vi "user32_BringWindowToTop.vi"(0 "hWnd":u32, 11 "错误输入（无错误）":errorcluster) -> (4 "dup hWnd":u32, 6 "success?":bool, 15 "错误输出":errorcluster)   [LabVIEW 2011]
doc: "该函数将指定的窗口设置到Z序的顶部。如果窗口为顶层窗口，则该窗口被激活；如果窗口为子窗口，则相应的顶级父窗口被激活。"
uses:
  user32.dll
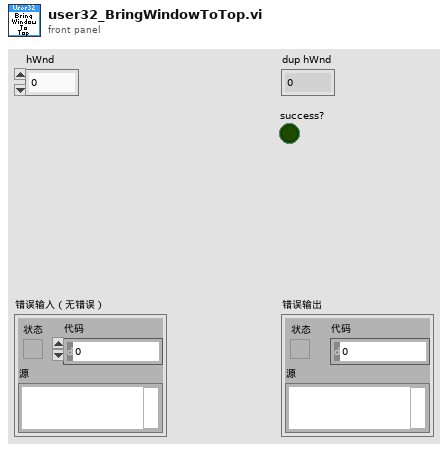
[diagram p1: front panel]
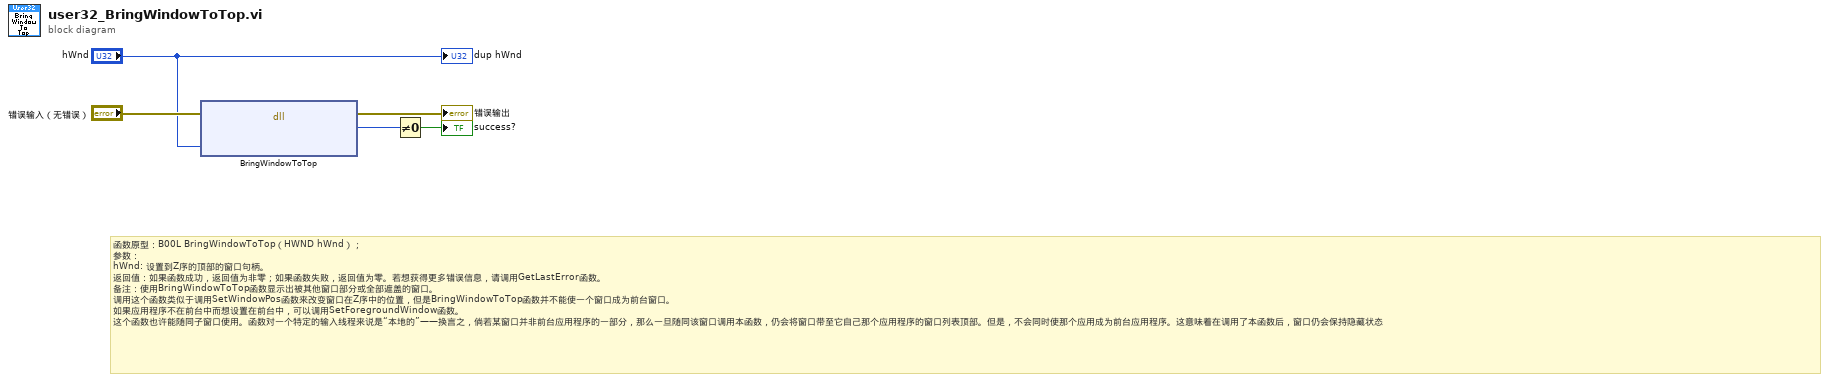
[diagram p0: block diagram]
diagram:
  # "函数原型：B00L BringWindowToTop（HWND hWnd）；\n参数：\nhWnd: 设置到Z序的顶部的窗口句柄。\n返回值：如果函数成功，返回值为非零；如果函数失败，返回值为零。若想获得更多错误信息，请调用GetLastError函数。\n备注：使用BringWindowToTop函数显示出被其他窗口部分或全部遮盖的窗口。\n调用这个函数类似于调用SetWindowPos函数来改变窗口在Z序中的位置，但是BringWindowToTop函数并不能使一个窗口成为前台窗口。\n如果应用程序不在前台中而想设置在前台中，可以调用SetForegroundWindow函数。\n这个函数也许能随同子窗口使用。函数对一个特定的输入线程来说是“本地的”——换言之，倘若某窗口并非前台应用程序的一部分，那么一旦随同该窗口调用本函数，仍会将窗口带至它自己那个应用程序的窗口列表顶部。但是，不会同时使那个应用成为前台应用程序。这意味着在调用了本函数后，窗口仍会保持隐藏状态"
  n1 = dll-call lib="user32.dll" fn="BringWindowToTop"(error in="错误输入（无错误）", "hWnd"="hWnd") -> (error out=→"错误输出":errorcluster, "bool"=w2:u8)  [unwired: 3 in, 1 out]
  n2 = Not Equal To 0?(x=w2) -> (x != 0?=→"success?":bool)
  "dup hWnd" <- "hWnd"
